vi "Read Network Master.vi"(8 "error in":errorcluster, 11 "Modbus master in":refnum<class "Modbus Master.lvclass">) -> (0 "error out":errorcluster, 2 "network master":refnum<class "Network Master.lvclass">, 3 "Modbus master out":refnum<class "Modbus Master.lvclass">)   [LabVIEW 2012, in "Modbus Master.lvclass"]
doc: "This VI is an accessor for the <B>network master</B> stored in the Modbus master instance. This accessor can be used as a property node. This network master is used by the Modbus instance to communicate on the physical bus."
uses:
  Modbus Master.lvclass
  Network Protocol/Network Master/Network Master.lvclass
  Modbus Master.lvclass/Modbus Master.ctl
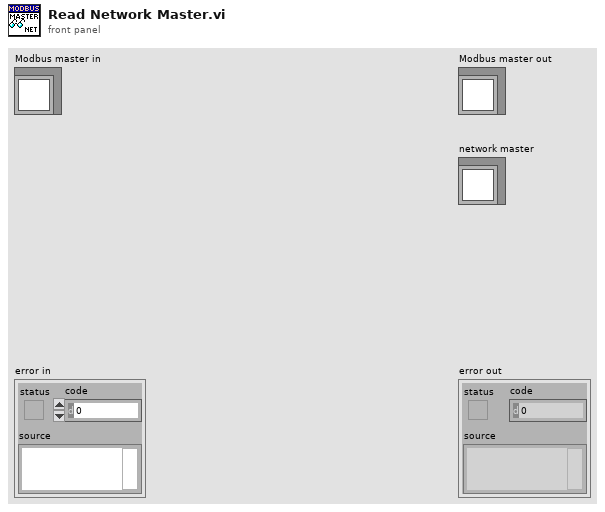
[diagram p1: front panel]
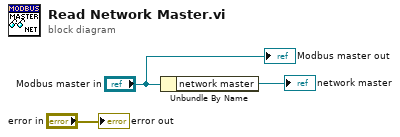
[diagram p0: block diagram]
diagram:
  n1 = Unbundle By Name("Modbus master in") -> ("network master"=→"network master":refnum<class "Network Master.lvclass">)
  "error out" <- "error in"
  "Modbus master out" <- "Modbus master in"
